vi "Etalon Setup Scanner.vi"() -> ()   [LabVIEW 2013]
panel:
  in  "GO Button":bool
  in  "Thin Step Size":i32=500
  in  "Thick Step Size":i32=100
  in  "Thick Lower Limit":i32=-5000
  in  "Thin Lower Limit":i32=-2000
  in  "Thick Upper Limit":i32=15000
  in  "Thin Upper Limit":i32=1500
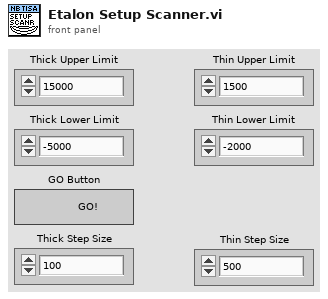
[diagram p1: front panel]
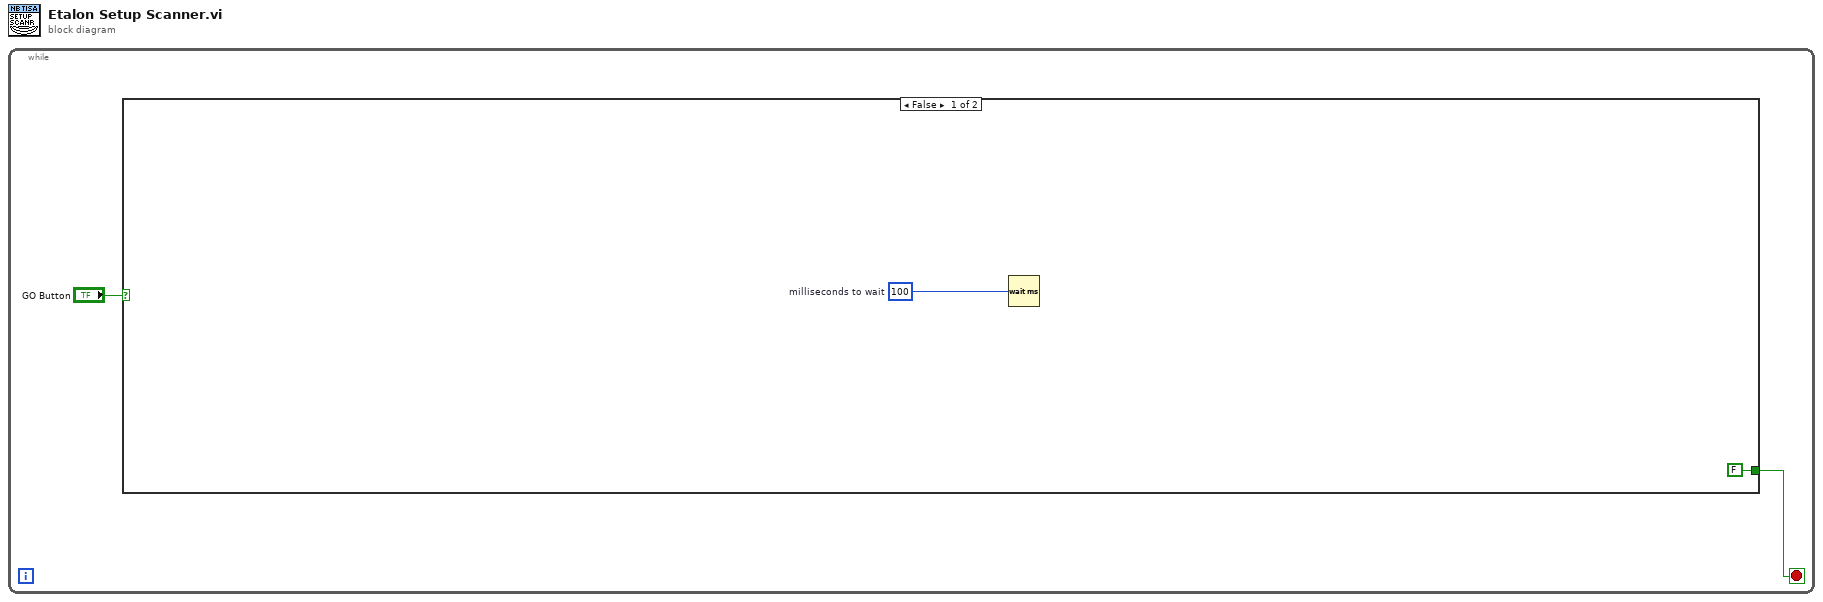
[diagram p0: block diagram]
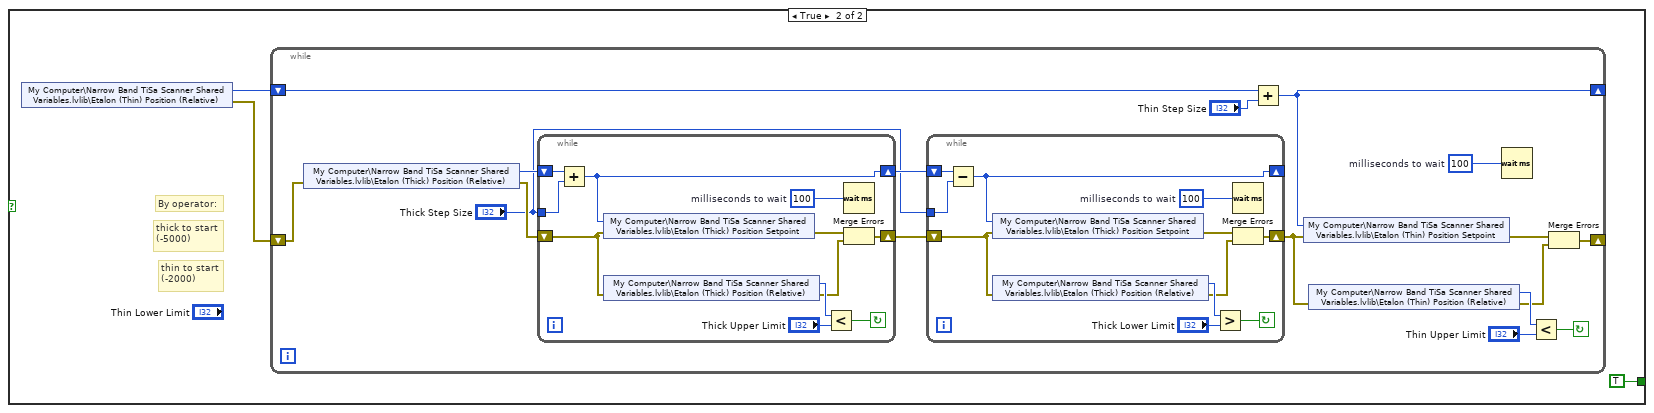
[diagram p2: hidden frame]
diagram:
  n1 = while {
    stop <- w1 stop-if-true
    n2 = case shown="False" "GO Button" {
      tunnel: [FALSE TRUE] -> w1
      frame False {
        w4 = u32 100  # milliseconds to wait
        n3 = Wait (ms)(milliseconds to wait=w4) -> ()  [unwired: 1 out]
      }
      frame True {
        # "By operator:"
        # "thin to start\n(-2000)"
        # "thick to start\n(-5000)"
        n4 = shared-variable "My Computer\\Narrow Band TiSa Scanner Shared Variables.lvlib\\Etalon (Thin) Position (Relative)"() -> (w6:i32, error out=w7:errorcluster)  [unwired: 1 in]
        n5 = while {
          shift-right: [w12] -> _
          shift-left: w6 -> [w15]
          shift-right: [w8] -> _
          shift-left: w7 -> [w16]
          stop <- w22 continue-if-true
          w9 = u32 100  # milliseconds to wait
          n6 = shared-variable "My Computer\\Narrow Band TiSa Scanner Shared Variables.lvlib\\Etalon (Thick) Position (Relative)"(error in=w16) -> (w21:i32, error out=w20:errorcluster)
          n7 = while {
            shift-right: [w41] -> w19
            shift-left: w21 -> [w43]
            tunnel: "Thick Step Size" -> [w42]
            shift-right: [w38] -> w18
            shift-left: w20 -> [w37]
            stop <- w44 continue-if-true
            w36 = u32 100  # milliseconds to wait
            n8 = Add(x=w43, y=w42) -> (x+y=w41:i32)
            n9 = shared-variable "My Computer\\Narrow Band TiSa Scanner Shared Variables.lvlib\\Etalon (Thick) Position Setpoint"(w41, error in=w37) -> (error out=w39:errorcluster)
            n10 = shared-variable "My Computer\\Narrow Band TiSa Scanner Shared Variables.lvlib\\Etalon (Thick) Position (Relative)"(error in=w37) -> (w46:i32, error out=w40:errorcluster)
            n11 = Less?(x=w46, y="Thick Upper Limit") -> (x < y?=w44:bool)
            n12 = Wait (ms)(milliseconds to wait=w36) -> ()  [unwired: 1 out]
            n13 = Merge Errors(w39, w40) -> (w38:errorcluster)
          }
          n14 = while {
            shift-right: [w31] -> _
            shift-left: w19 -> [w33]
            tunnel: "Thick Step Size" -> [w32]
            shift-right: [w28] -> w13
            shift-left: w18 -> [w27]
            stop <- w34 continue-if-true
            w25 = u32 100  # milliseconds to wait
            n15 = Subtract(x=w33, y=w32) -> (x-y=w31:i32)
            n16 = shared-variable "My Computer\\Narrow Band TiSa Scanner Shared Variables.lvlib\\Etalon (Thick) Position Setpoint"(w31, error in=w27) -> (error out=w29:errorcluster)
            n17 = shared-variable "My Computer\\Narrow Band TiSa Scanner Shared Variables.lvlib\\Etalon (Thick) Position (Relative)"(error in=w27) -> (w35:i32, error out=w30:errorcluster)
            n18 = Greater?(x=w35, y="Thick Lower Limit") -> (0:w34:bool)
            n19 = Wait (ms)(milliseconds to wait=w25) -> ()  [unwired: 1 out]
            n20 = Merge Errors(w29, w30) -> (w28:errorcluster)
          }
          n21 = Add(x=w15, y="Thin Step Size") -> (x+y=w12:i32)
          n22 = shared-variable "My Computer\\Narrow Band TiSa Scanner Shared Variables.lvlib\\Etalon (Thin) Position Setpoint"(w12, error in=w13) -> (error out=w11:errorcluster)
          n23 = shared-variable "My Computer\\Narrow Band TiSa Scanner Shared Variables.lvlib\\Etalon (Thin) Position (Relative)"(error in=w13) -> (w24:i32, error out=w10:errorcluster)
          n24 = Wait (ms)(milliseconds to wait=w9) -> ()  [unwired: 1 out]
          n25 = Less?(x=w24, y="Thin Upper Limit") -> (x < y?=w22:bool)
          n26 = Merge Errors(w11, w10) -> (w8:errorcluster)
        }
      }
    }
  }
